vi "Get Wavelengths.vi"(7 "Calibration File":path=path "C:/Users/Michael/Documents/GitHub/CampenLab/data/calib_1.csv", 8 "X Binning":i32, 9 "X Length":i32, 10 "X Start":i32, 11 "Spectrometer Wavelength":dbl) -> (2 "wavelengths":dbl[](array[numeric]) format="%#_10g")   [LabVIEW 2020, in "Spectrometer Calibration.lvlib"]
uses:
  Spectrometer Calibration.lvlib
  <vilib>/Analysis/1siggen.llb/Ramp Pattern by Samples.vi
  <vilib>/Analysis/NI_AALBase.lvlib
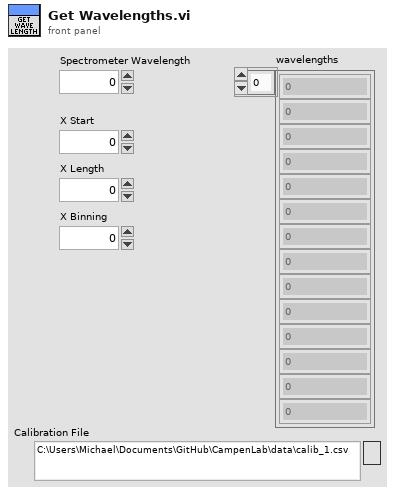
[diagram p1: front panel]
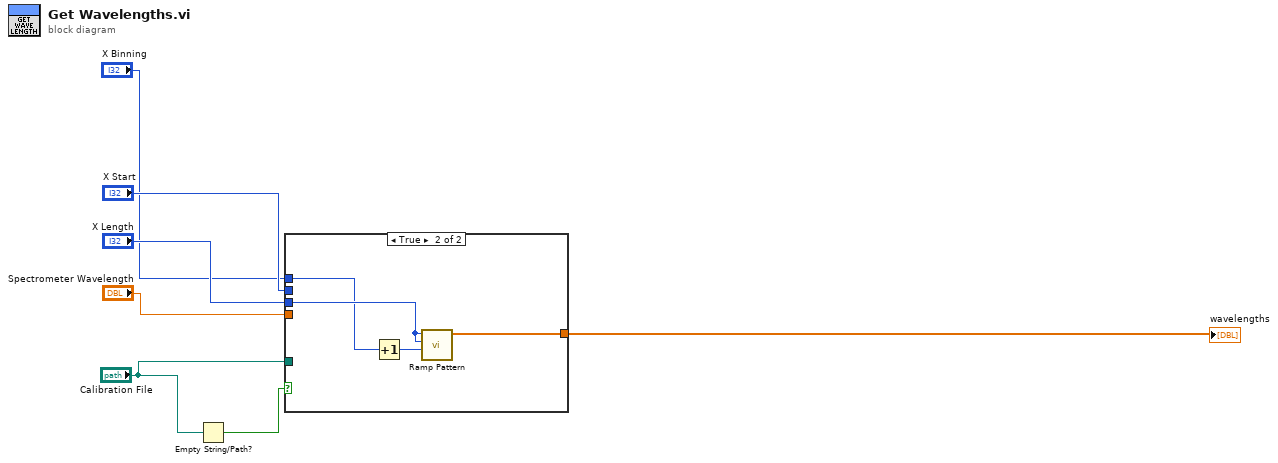
[diagram p0: block diagram]
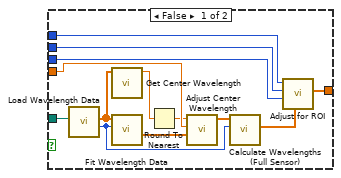
[diagram p2: hidden frame]
diagram:
  n1 = Empty String/Path?(string/path="Calibration File") -> (empty?=w1:bool)
  n2 = case shown="True" w1 {
    tunnel: "Spectrometer Wavelength" -> [w18 _]
    tunnel: "X Start" -> [w12 _]
    tunnel: [w11 w21] -> w5
    tunnel: "X Length" -> [w10 w24]
    tunnel: "X Binning" -> [w9 w23]
    tunnel: "Calibration File" -> [w8 _]
    frame False {
      n3 = call "Load Wavelength Data.vi"("Calibration File"=w8) -> ("Numeric"=w14:i32, "Array"=w20:dbl[])  [unwired: 8 in, 1 out]
      n4 = call "Get Center Wavelength.vi"("Array"=w20) -> ("center wavelength"=w19:dbl)  [unwired: 9 in, 1 out]
      n5 = call "Fit Wavelength Data.vi"("Numeric"=w14, "Array"=w20) -> ("Polynomial Coefficients"=w16:dbl[])  [unwired: 7 in, 2 out]
      n6 = Round To Nearest(number=w19) -> (nearest integer value=w17:dbl)
      n7 = call "Adjust Center Wavelength.vi"("Polynomial Coefficients in"=w16, "Spectrometer Wavelength"=w18, "Numeric"=w17) -> ("Polynomial Coefficients out"=w15:dbl[])  [unwired: 8 in]
      n8 = call "Calculate Wavelengths (Full Sensor).vi"("Numeric"=w14, "Polynomial Coefficients in"=w15) -> ("wavelengths"=w13:dbl[])  [unwired: 8 in, 1 out]
      n9 = call "Adjust for ROI.vi"("wavelengths"=w13, "X Length"=w10, "X Start"=w12, "X Binning"=w9) -> ("Wavelengths"=w11:dbl[])  [unwired: 5 in, 2 out]
    }
    frame True {
      n10 = Increment(x=w23) -> (x+1=w22:i32)
      n11 = call-poly <vilib>:"Ramp Pattern.vi"("start"=w22, "end"=w24, "samples"=w24) -> ("Ramp Pattern"=w21:dbl[])  [unwired: 7 in, 1 out]
    }
  }
  "wavelengths" <- w5
